vi "ToRepo.vi"(8 "error in":errorcluster, 9 "to repo cluster":T1, 10 "repository in":refnum<class "NISE_CEF_Repository.lvclass">, 11 "node in":refnum<class "VI modification collection.lvclass">) -> (0 "error out":errorcluster, 2 "repository out":refnum<class "NISE_CEF_Repository.lvclass">, 3 "node out":refnum<class "VI modification collection.lvclass">)   [LabVIEW 2013, in "VI modification collection.lvclass"]
doc: "Transfers the information from the tree node into the repo. How it is stored in the repo depends on the Repo."
uses:
  VI modification collection.lvclass
  <vilib>/NI/Configuration Framework/Repository/NISE_CEF_Repository.lvclass
  <vilib>/NI/Configuration Framework/Node/ToRepoCluster.ctl
  Modifier UI/modification container/modification container.lvclass
  Modifier UI/modification container/modification container.lvclass/modification container.ctl
  Modifier UI/modification container/Write mods.vi
  <vilib>/NI/Configuration Framework/Node/NISE_CEF_Node.lvclass
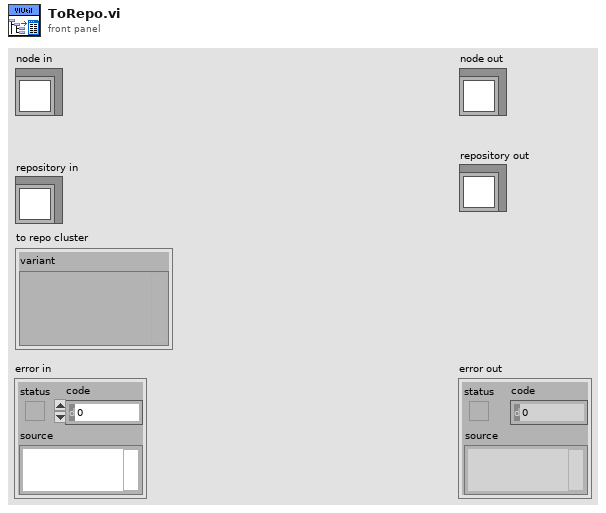
[diagram p1: front panel]
types:
  T1 = typedef "NISE_CEF_Node.lvclass/ToRepoCluster.ctl" = cluster{"variant":variant}
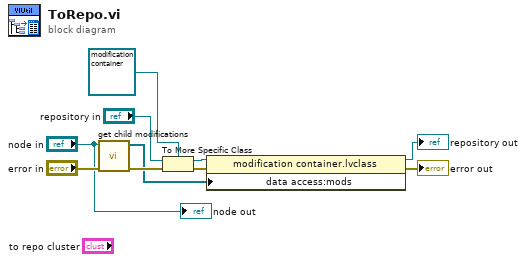
[diagram p0: block diagram]
diagram:
  n1 = call "get child modifications.vi"("error in"="error in", "VI modification collection in"="node in") -> ("error out"=w3:errorcluster, "modifications"=w2:refnum<class "VI modification.lvclass">[])  [unwired: 8 in]
  n2 = To More Specific Class(target class=refnum<class "modification container.lvclass"> refnum ("modification container.lvclass"), reference="repository in", error in=w3) -> (specific class reference=w5:refnum<class "modification container.lvclass">, error out=w7:errorcluster)
  n3 = property class="modification container.lvclass"(reference=w5, error in=w7, "data access:mods"=w2) -> (reference out=→"repository out":refnum<class "modification container.lvclass">, error out=→"error out":errorcluster)
  "node out" <- "node in"
